vi "Fuzzy_Input.vi"() -> ()   [LabVIEW 2016]
panel:
  in  "stop":bool
  in  "Membership Function 3":dbl[](array[numeric])
  in  "Membership Function 2":dbl[](array[numeric])
  in  "Membership Function 1":dbl[](array[numeric])
  out "XY Graph":cluster{"Array":dbl[], dbl[]}[](graph)
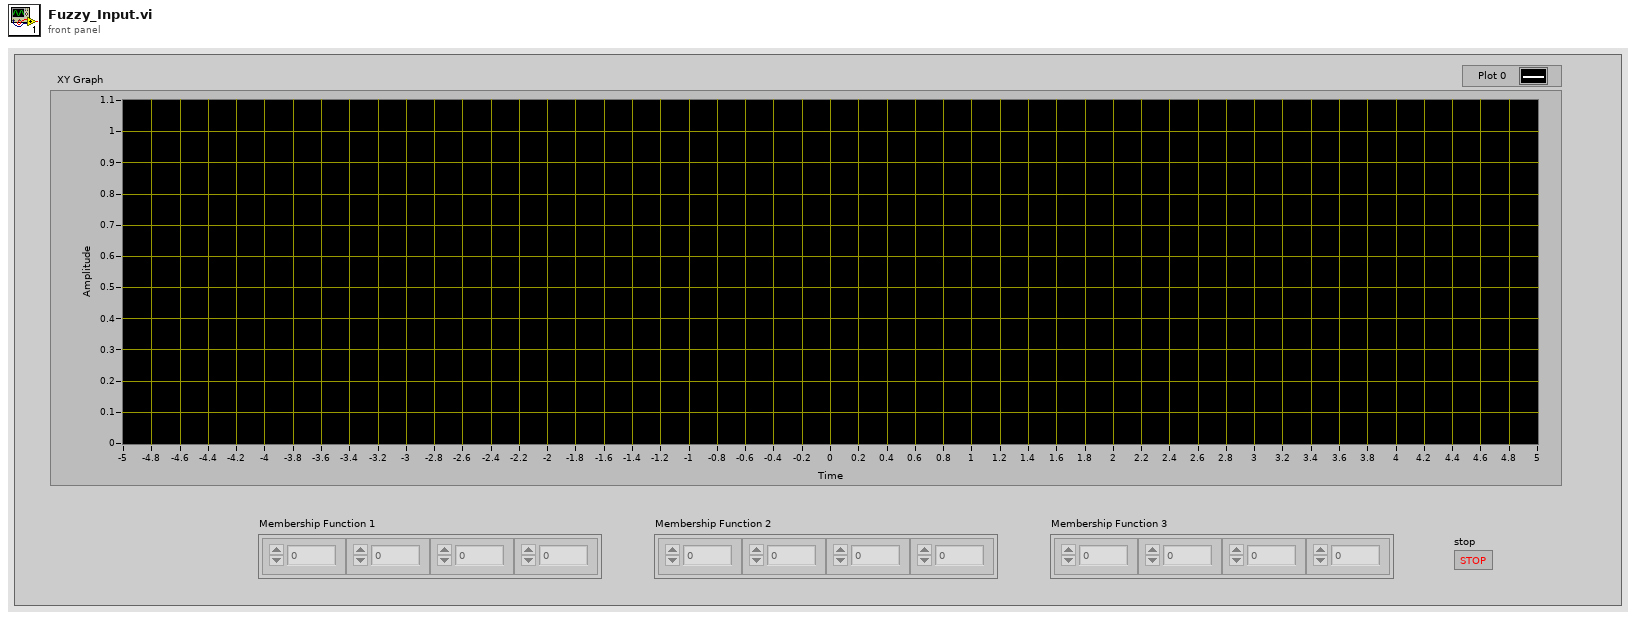
[diagram p1: front panel]
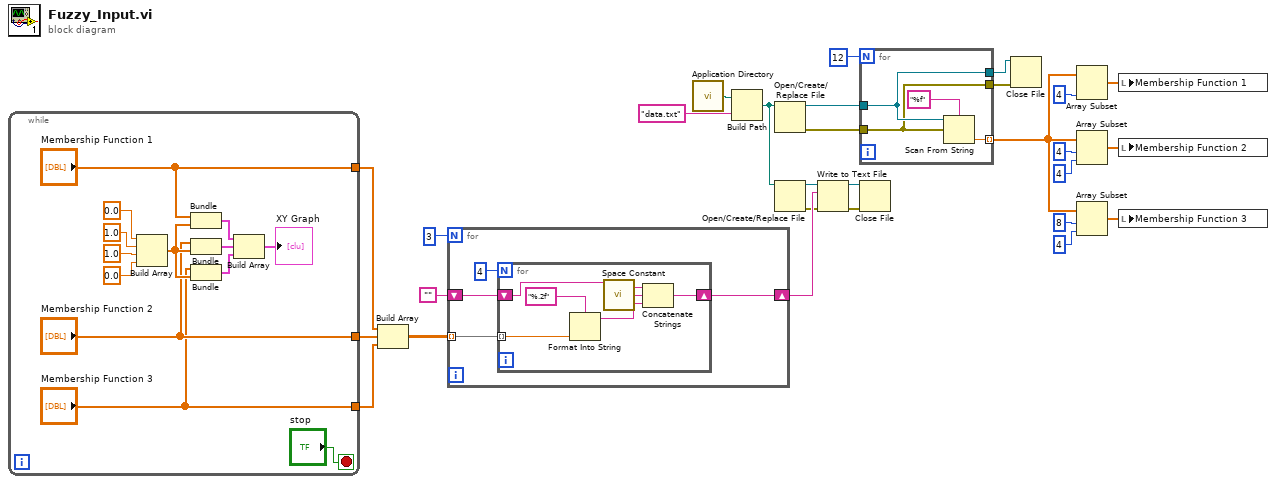
[diagram p0: block diagram]
diagram:
  n1 = while {
    tunnel: ["Membership Function 1"] -> w12
    tunnel: ["Membership Function 2"] -> w11
    tunnel: ["Membership Function 3"] -> w10
    stop <- "stop" stop-if-true
    n2 = Build Array(0.0 ("element"), 1.0 ("element"), 1.0 ("element"), 0.0 ("element")) -> (w33:dbl[])
    n3 = Bundle("Membership Function 1"="Membership Function 1", w33) -> (w41:cluster{"Membership Function 1":dbl[], dbl[]})  [unwired: 1 in]
    n4 = Bundle("Membership Function 2"="Membership Function 2", w33) -> (w40:cluster{"Membership Function 2":dbl[], dbl[]})  [unwired: 1 in]
    n5 = Bundle("Membership Function 3"="Membership Function 3", w33) -> (w39:cluster{"Membership Function 3":dbl[], dbl[]})  [unwired: 1 in]
    n6 = Build Array(w41, w40, w39) -> (→"XY Graph":cluster{"Membership Function 3":dbl[], dbl[]}[])
  }
  n7 = Build Array(w12, w11, w10) -> (w7:dbl[][])
  n8 = for {
    N: 3 -> [_]
    tunnel: w7 -> [w44] mode=indexing
    shift-right: [w43] -> w5
    shift-left: "" -> [w42]
    n9 = for {
      N: 4 -> [_]
      tunnel: w44 -> [w50] mode=indexing
      shift-right: [w49] -> w43
      shift-left: w42 -> [w48]
      n10 = Format Into String(format string="%.2f", w50) -> (resulting string=w46:string)  [unwired: 2 in, 1 out]
      n11 = call <vilib>:"Space Constant.vi"() -> ("String"=w47:string)
      n12 = Concatenate Strings(w48, w47, w46) -> (w49:string)
    }
  }
  n13 = call <vilib>:"Application Directory.vi"() -> ("Application Directory"=w27:path)
  n14 = Build Path(base path=w27, name or relative path="data.txt") -> (appended path=w8:path)
  n15 = Open/Create/Replace File(file path (use dialog)=w8) -> (refnum out=w25:refnum<file>, error out=w24:errorcluster)  [unwired: 5 in, 1 out]
  n16 = Open/Create/Replace File(file path (use dialog)=w8) -> (refnum out=w4:refnum<file>, error out=w3:errorcluster)  [unwired: 5 in, 1 out]
  n17 = Write to Text File(file (use dialog)=w4, text=w5, error in=w3) -> (refnum out=w2:refnum<file>, error out=w1:errorcluster)  [unwired: 1 in, 1 out]
  n18 = for {
    N: 12 -> [_]
    tunnel: w25 -> [w53]
    tunnel: w24 -> [w52]
    tunnel: [w54] -> w17 mode=indexing
    tunnel: [w53] -> w14
    tunnel: [w52] -> w13
    n19 = Scan From String("%f" ("format string"), w53, w52) -> (output 1=w54:dbl)  [unwired: 1 in, 2 out]
  }
  n20 = Close File(refnum=w2, error in=w1) -> ()  [unwired: 2 out]
  n21 = Close File(refnum=w14, error in=w13) -> ()  [unwired: 2 out]
  n22 = Array Subset(array=w17, length=4) -> (w22:dbl[])  [unwired: 1 in]
  n23 = Array Subset(array=w17, index=4, length=4) -> (w21:dbl[])
  n24 = Array Subset(array=w17, index=8, length=4) -> (w18:dbl[])
  n25 = local write "Membership Function 1"(w22) -> ()
  n26 = local write "Membership Function 2"(w21) -> ()
  n27 = local write "Membership Function 3"(w18) -> ()
